vi "LV10_2.vi"() -> ()   [LabVIEW 2016]
uses:
  <vilib>/picture/picture.llb/Draw 8-Bit Pixmap.vi
  <vilib>/imath/engines/lvmath2/RunTimeEngine/BuiltInFunctions/fft2d/NIMS_fft2d.vi
  <instcachedir>/0/NIMS_fft2d_01A33FFC48FF4786A19C9A8A715D9BC4.lvgen/NIMS_fft2d_01A33FFC48FF4786A19C9A8A715D9BC4_000.vi
  <vilib>/imath/engines/lvmath2/RunTimeEngine/BuiltInFunctions/fftshift/NIMS_fftshift(GM).vi
  <instcachedir>/0/NIMS_fftshift(GM)_854644D58B904BE68890FF38C728418A.lvgen/NIMS_fftshift(GM)_854644D58B904BE68890FF38C728418A_003.vi
  <vilib>/imath/engines/lvmath2/RunTimeEngine/BuiltInFunctions/abs/NIMS_abs(signed).vi
  <instcachedir>/0/NIMS_abs(signed)_C4FCB8E6058B49B797C7C8D53CA5F6EC.lvgen/NIMS_abs(signed)_C4FCB8E6058B49B797C7C8D53CA5F6EC_003.vi
  <vilib>/imath/engines/lvmath2/RunTimeEngine/ErrorHandling/NIMS_Error From Error Code.vi
  <vilib>/imath/engines/lvmath2/RunTimeEngine/BuiltInFunctions/size/NIMS_I32Row=size(GM).vi
  <instcachedir>/0/NIMS_I32Row=size(GM)_10ACDCB9F1F84A7E9F42C91D87611FB5.lvgen/NIMS_I32Row=size(GM)_10ACDCB9F1F84A7E9F42C91D87611FB5_006.vi
  <vilib>/imath/engines/lvmath2/RunTimeEngine/IndexRead/NIMS V(S).vi
  <instcachedir>/0/NIMS V(S)_0488751826AF41519A22953C041130DC.lvgen/NIMS V(S)_0488751826AF41519A22953C041130DC_002.vi
  <vilib>/imath/engines/lvmath2/RunTimeEngine/BuiltInFunctions/round/NIMS_round(DBL-S).vi
  <vilib>/imathl/engines/lvmath/Functions/Error Handling/Create Error.vi
  <vilib>/imath/engines/lvmath2/RunTimeEngine/BuiltInFunctions/randnormal/NIMS_randnormal(I32,I32).vi
  <vilib>/imath/engines/lvmath2/RunTimeEngine/ArithmeticOperatorToken/NIMS_ArithmeticOperator_plus.vi
  <instcachedir>/0/NIMS_ArithmeticOperator_plus_0120E0498A0F4B4B9BDCAC2554767A4E.lvgen/NIMS_ArithmeticOperator_plus_0120E0498A0F4B4B9BDCAC2554767A4E_012.vi
  <vilib>/imath/engines/lvmath2/RunTimeEngine/RangeToken/NIMS_Range.vi
  <instcachedir>/0/NIMS_Range_A7C094595B484CA7AF10685B02D808ED.lvgen/NIMS_Range_A7C094595B484CA7AF10685B02D808ED_000.vi
  <vilib>/imath/engines/lvmath2/RunTimeEngine/IndexReplace/NIMS M(V,$)=S.vi
  <instcachedir>/0/NIMS M(V,$)=S_90089C354C3E453AB2EA93F9AE4B1AFC.lvgen/NIMS M(V,$)=S_90089C354C3E453AB2EA93F9AE4B1AFC_000.vi
  <vilib>/imath/engines/lvmath2/RunTimeSupport/NIMS_Error if Not Equal.vi
  <instcachedir>/0/NIMS_Error if Not Equal_43252A79AD05436189442EC0C5E5AB8A.lvgen/NIMS_Error if Not Equal_43252A79AD05436189442EC0C5E5AB8A_001.vi
  <vilib>/imath/engines/lvmath2/RunTimeEngine/ErrorHandling/NIMS_Create Error From Enums.vi
  <vilib>/imath/engines/lvmath2/RunTimeEngine/IndexReplace/NIMS M($,V)=S.vi
  <instcachedir>/0/NIMS M($,V)=S_8FF4B0FF94A24B3598424F2A899DBD06.lvgen/NIMS M($,V)=S_8FF4B0FF94A24B3598424F2A899DBD06_000.vi
  <vilib>/imath/engines/lvmath2/RunTimeEngine/BuiltInFunctions/ifft2d/NIMS_ifft2d.vi
  <vilib>/imath/engines/lvmath2/RunTimeEngine/NodeEndStatement/NIMS_NodeEndStatement_Output.vi
  <instcachedir>/0/NIMS_NodeEndStatement_Output_53EC0D466D134D7ABD903AC30B43404B.lvgen/NIMS_NodeEndStatement_Output_53EC0D466D134D7ABD903AC30B43404B_003.vi
  <instcachedir>/0/NIMS_NodeEndStatement_Output_53EC0D466D134D7ABD903AC30B43404B.lvgen/NIMS_NodeEndStatement_Output_53EC0D466D134D7ABD903AC30B43404B_002.vi
  <vilib>/imath/engines/lvmath2/RunTimeEngine/ErrorHandling/NIMS_Finalize Error.vi
panel:
  in  "Lowpass cutoff = K (*p)":dbl(slide) scale=0.01..1.0
  in  "Noise level":dbl(slide) scale=0.0..100.0
  out "Noisy image":picture
  out "Filtered image spectrum":dbl[][](graph)
  out "Noisy image spectrum":dbl[][](graph)
  out "Original image spectrum":dbl[][](graph)
  out "Original image":picture
  in  "Stop Button":bool
  out "Filtered image":picture
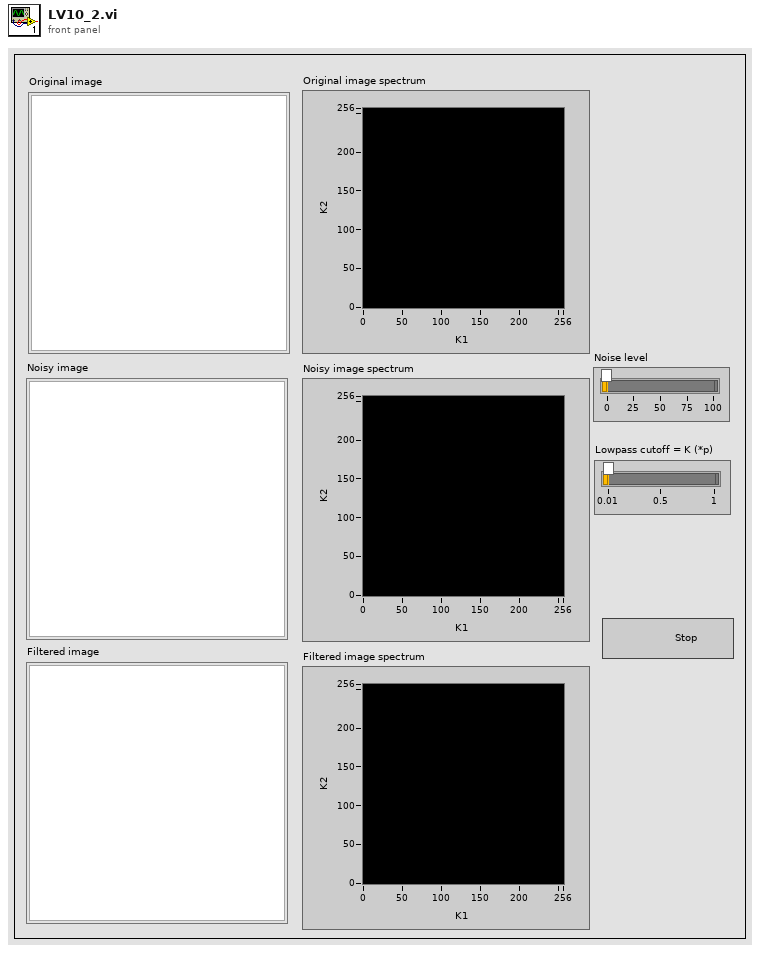
[diagram p1: front panel]
types:
  T1 = typedef "imagedata.ctl" = cluster{"image type":i32, "image depth":i32, "image":u8[], "mask":u8[], "colors":u32[], "Rectangle":cluster{"left":i16, "top":i16, "right":i16, "bottom":i16}}
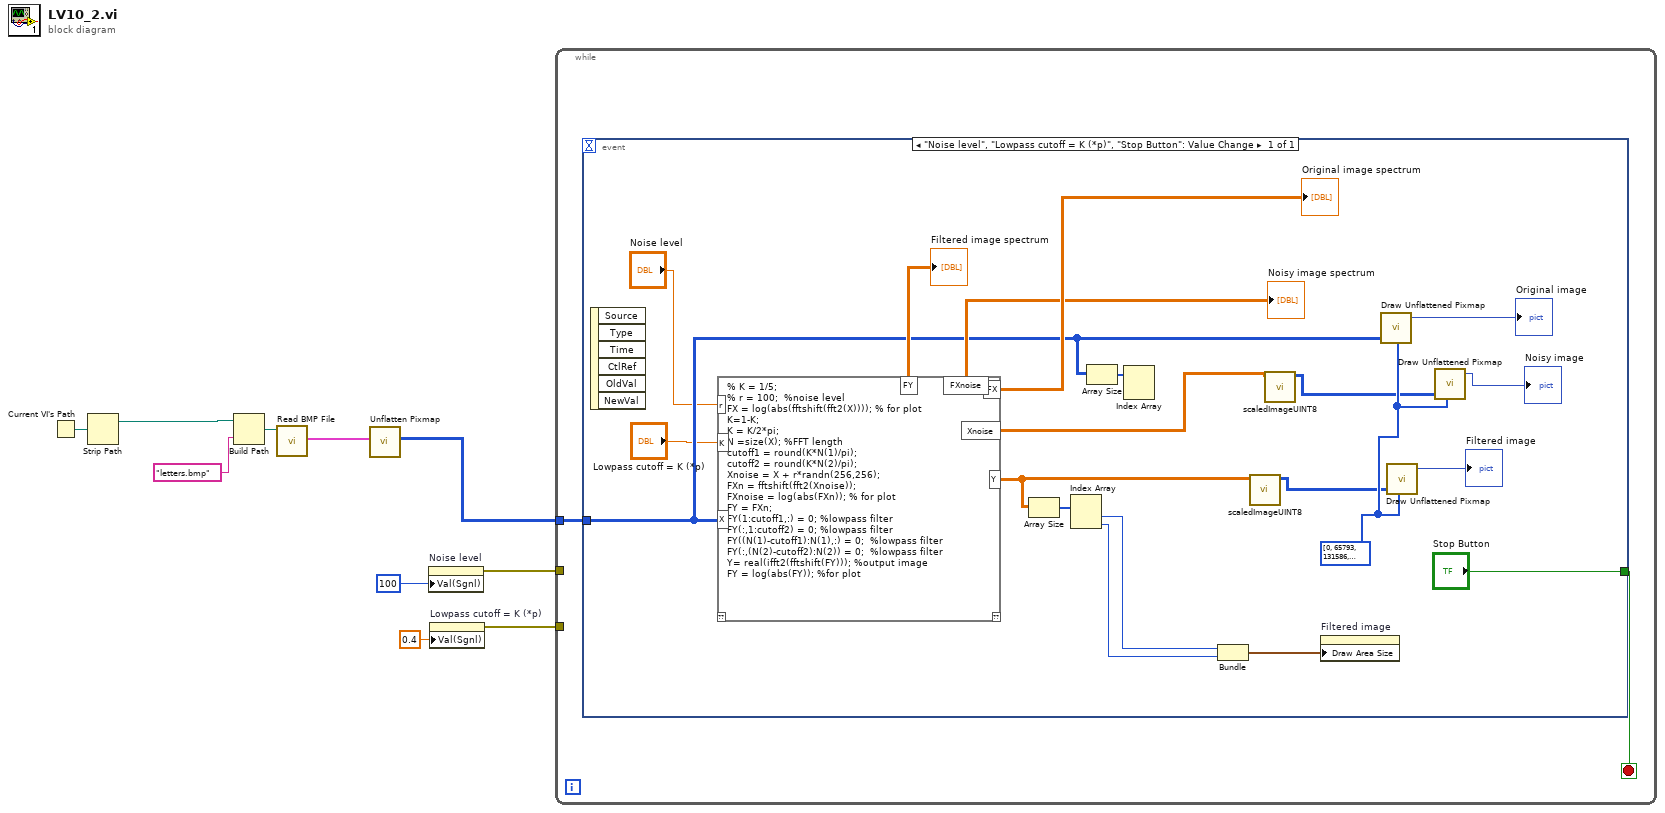
[diagram p0: block diagram]
diagram:
  n1 = Current VI's Path() -> (path=w10:path)
  n2 = Strip Path(path=w10) -> (stripped path=w1:path)  [unwired: 1 out]
  n3 = Build Path(base path=w1, name or relative path="letters.bmp") -> (appended path=w7:path)
  n4 = call <vilib>:"Read BMP File.vi"("path to BMP file"=w7) -> ("image data"=w8:T1)  [unwired: 8 in, 2 out]
  n5 = call <vilib>:"Unflatten Pixmap.vi"("image data"=w8) -> ("8-bit pixmap"=w6:u8[][])  [unwired: 4 in, 6 out]
  n6 = property on="Noise level" class="Slide (strict)"("Val(Sgnl)"=100 ("Value (Signaling)")) -> (error out=w5:errorcluster)  [unwired: 2 in, 1 out]
  n7 = property on="Lowpass cutoff = K (*p)" class="Slide (strict)"("Val(Sgnl)"=0.4 ("Value (Signaling)")) -> (error out=w3:errorcluster)  [unwired: 2 in, 1 out]
  n8 = while {
    tunnel: w6 -> [w11]
    tunnel: w5 -> [_]
    tunnel: w3 -> [_]
    stop <- w12 stop-if-true
    n9 = event shown="[0] \"Noise level\", \"Lowpass cutoff = K (*p)\", \"Stop Button\": Value Change" {
      selector: _ -> [_]
      dyn-events: _ -> [_]
      timeout: _ -> [_]
      tunnel: ["Stop Button"] -> w12
      tunnel: w11 -> [w23]
      event "Noise level", "Lowpass cutoff = K (*p)", "Stop Button": Value Change {
        w20 = u32[] [0, 65793, 131586, 197379, 263172, 328965, 394758, 460551, 526344, 592137, 657930, 723723, 789516, 855309, 921102, 986895, 1052688, 1118481, 1184274, 1250067, 1315860, 1381653, 1447446, 1513239, 1579032, 1644825, 1710618, 1776411, 1842204, 1907997, 1973790, 2039583, 2105376, 2171169, 2236962, 2302755, 2368548, 2434341, 2500134, 2565927, 2631720, 2697513, 2763306, 2829099, 2894892, 2960685, 3026478, 3092271, 3158064, 3223857, 3289650, 3355443, 3421236, 3487029, 3552822, 3618615, 3684408, 3750201, 3815994, 3881787, 3947580, 4013373, 4079166, 4144959, 4210752, 4276545, 4342338, 4408131, 4473924, 4539717, 4605510, 4671303, 4737096, 4802889, 4868682, 4934475, 5000268, 5066061, 5131854, 5197647, 5263440, 5329233, 5395026, 5460819, 5526612, 5592405, 5658198, 5723991, 5789784, 5855577, 5921370, 5987163, 6052956, 6118749, 6184542, 6250335, 6316128, 6381921, 6447714, 6513507, 6579300, 6645093, 6710886, 6776679, 6842472, 6908265, 6974058, 7039851, 7105644, 7171437, 7237230, 7303023, 7368816, 7434609, 7500402, 7566195, 7631988, 7697781, 7763574, 7829367, 7895160, 7960953, 8026746, 8092539, 8158332, 8224125, 8289918, 8355711, 8421504, 8487297, 8553090, 8618883, 8684676, 8750469, 8816262, 8882055, 8947848, 9013641, 9079434, 9145227, 9211020, 9276813, 9342606, 9408399, 9474192, 9539985, 9605778, 9671571, 9737364, 9803157, 9868950, 9934743, 10000536, 10066329, 10132122, 10197915, 10263708, 10329501, 10395294, 10461087, 10526880, 10592673, 10658466, 10724259, 10790052, 10855845, 10921638, 10987431, 11053224, 11119017, 11184810, 11250603, 11316396, 11382189, 11447982, 11513775, 11579568, 11645361, 11711154, 11776947, 11842740, 11908533, 11974326, 12040119, 12105912, 12171705, 12237498, 12303291, 12369084, 12434877, 12500670, 12566463, 12632256, 12698049, 12763842, 12829635, 12895428, 12961221, 13027014, 13092807, 13158600, 13224393, 13290186, 13355979, 13421772, 13487565, 13553358, 13619151, 13684944, 13750737, 13816530, 13882323, 13948116, 14013909, 14079702, 14145495, 14211288, 14277081, 14342874, 14408667, 14474460, 14540253, 14606046, 14671839, 14737632, 14803425, 14869218, 14935011, 15000804, 15066597, 15132390, 15198183, 15263976, 15329769, 15395562, 15461355, 15527148, 15592941, 15658734, 15724527, 15790320, 15856113, 15921906, 15987699, 16053492, 16119285, 16185078, 16250871, 16316664, 16382457, 16448250, 16514043, 16579836, 16645629, 16711422, 16777215] ("colors")
        n10 = event-data() -> ()  [unwired: 1 in, 6 out]
        n11 = mathscript code="% K = 1/5;\n% r = 100;  %noise level\nFX = log(abs(fftshift(fft2(X)))); % for plot\nK=1-K;\nK = K/2*pi;\nN =size(X); %FFT length\ncutoff1 = round(K*N(1)/pi); \ncutoff2 = round(K*N(2)/pi); \nXnoise = X + r*randn(256,256);\nFXn = fftshift(fft2(Xnoise));\nFXnoise = log(abs(FXn)); % for plot\nFY = FXn;\nFY(1:cutoff1,:) = 0; %lowpass filter\nFY(:,1:cutoff2) = 0; %lowpass filter\nFY((N(1)-cutoff1):N(1),:) = 0;  %lowpass filter\nFY(:,(N(2)-cutoff2):N(2)) = 0;  %lowpass filter\nY= real(ifft2(fftshift(FY))); %output image\nFY = log(abs(FY)); %for plot"("X"=w23, "r"="Noise level", "K"="Lowpass cutoff = K (*p)") -> ("Y"=w25:dbl[][], "FX"=→"Original image spectrum":cdb[][], "Xnoise"=w14:dbl[][], "FXnoise"=→"Noisy image spectrum":cdb[][], "FY"=→"Filtered image spectrum":cdb[][])  [unwired: 1 in, 1 out]
        n12 = Array Size(array=w25) -> (size(s)=w24:i32[])
        n13 = Index Array(array=w24) -> (element #1=w21:i32, element #2=w18:i32)  [unwired: 2 in]
        n14 = Array Size(array=w23) -> (size(s)=w22:i32[])
        n15 = Index Array(array=w22) -> ()  [unwired: 2 in, 2 out]
        n16 = Bundle(w21, w18) -> (w32:cluster{i32, i32})  [unwired: 1 in]
        n17 = call "scaledImageUINT8.vi"("double image"=w25) -> ("uint8 image"=w17:u8[][])  [unwired: 10 in]
        n18 = call "scaledImageUINT8.vi"("double image"=w14) -> ("uint8 image"=w13:u8[][])  [unwired: 10 in]
        n19 = property on="Filtered image" class="Pict"("Draw Area Size"=w32) -> ()  [unwired: 2 in, 2 out]
        n20 = call-poly <vilib>:"Draw Unflattened Pixmap.vi"("data"=w23, "color table"=w20) -> ("new picture"=→"Original image":picture)  [unwired: 7 in]
        n21 = call-poly <vilib>:"Draw Unflattened Pixmap.vi"("data"=w17, "color table"=w20) -> ("new picture"=→"Filtered image":picture)  [unwired: 7 in]
        n22 = call-poly <vilib>:"Draw Unflattened Pixmap.vi"("data"=w13, "color table"=w20) -> ("new picture"=→"Noisy image":picture)  [unwired: 7 in]
      }
    }
  }
